vi "make_tilt_stage_array (SubVI).vi"(1 "Tilt settings":T1={"thetaY steps"=0.0, "thetaZ steps"=6.0, "Run thetaY?"=FALSE, "Run thetaZ?"=FALSE, "# repeats \n   in thetaY"=0, "# repeats \n   in thetaZ"=0}) -> (0 "Tot Stage Arr":dbl[][](array[numeric]))   [LabVIEW 2016]
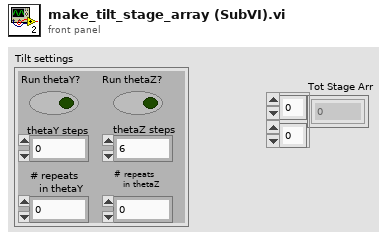
[diagram p1: front panel]
types:
  T1 = cluster{"thetaY steps":dbl, "thetaZ steps":dbl, "Run thetaY?":bool, "Run thetaZ?":bool, "# repeats \n   in thetaY":i32, "# repeats \n   in thetaZ":i32}
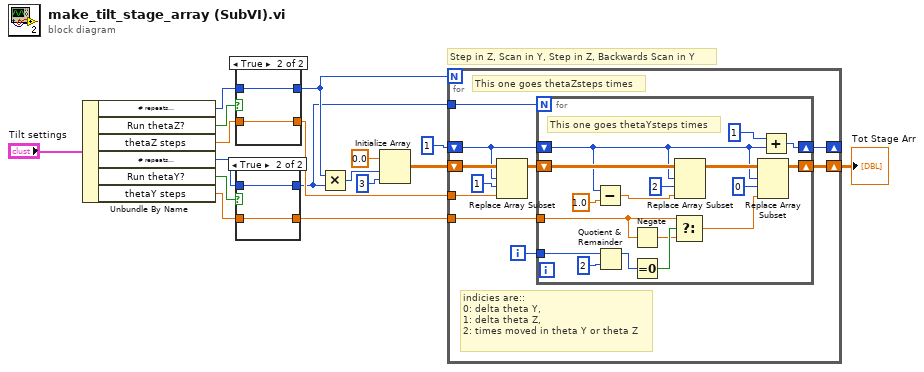
[diagram p0: block diagram]
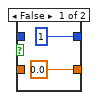
[diagram p2: hidden frame]
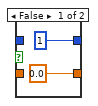
[diagram p3: hidden frame]
diagram:
  # "Step in Z, Scan in Y, Step in Z, Backwards Scan in Y"
  n1 = Unbundle By Name("Tilt settings") -> ("# repeats \n   in thetaZ"=w6:i32, "Run thetaZ?"=w5:bool, "thetaZ steps"=w4:dbl, "# repeats \n   in thetaY"=w9:i32, "Run thetaY?"=w8:bool, "thetaY steps"=w7:dbl)
  n2 = case shown="True" w5 {
    tunnel: w4 -> [_ w20]
    tunnel: w6 -> [_ w21]
    tunnel: [1 ("# steps to\nend thetaY") w21] -> w3
    tunnel: [0.0 ("end thetaZ") w20] -> w12
    frame False {
    }
    frame True {
    }
  }
  n3 = case shown="True" w8 {
    tunnel: w7 -> [_ w24]
    tunnel: w9 -> [_ w25]
    tunnel: [1 ("# steps to\nend thetaY") w25] -> w2
    tunnel: [0.0 ("end thetaZ") w24] -> w11
    frame False {
    }
    frame True {
    }
  }
  n4 = Multiply(x=w3, y=w2) -> (x*y=w1:i32)
  n5 = Initialize Array(0.0 ("element"), w1, 3 ("dimension size")) -> (w10:dbl[][])
  n6 = for {
    N: w3 -> [_]
    tunnel: w11 -> [w35]
    shift-right: [w27] -> _
    shift-left: 1 -> [w29]
    tunnel: w12 -> [w33]
    tunnel: w2 -> [w31]
    shift-right: [w32] -> w13
    shift-left: w10 -> [w30]
    i -> [w28]
    # "indicies are:: \n0: delta theta Y, \n1: delta theta Z, \n2: times moved in theta Y or theta Z"
    # "This one goes thetaZsteps times"
    n7 = Replace Array Subset(array=w30, new element=w33, index (row)=w29, index (col)=1 ("disabled index (col)")) -> (w26:dbl[][])
    n8 = for {
      N: w31 -> [_]
      tunnel: w35 -> [w46]
      tunnel: w28 -> [w45]
      shift-right: [w40] -> w27
      shift-left: w29 -> [w36]
      shift-right: [w44] -> w32
      shift-left: w26 -> [w42]
      # "This one goes thetaYsteps times"
      n9 = Subtract(x=w36, y=1.0) -> (x-y=w38:dbl)
      n10 = Quotient & Remainder(x=w45, y=2) -> (x-y*floor(x/y)=w50:i32)  [unwired: 1 out]
      n11 = Negate(x=w46) -> (-x=w47:dbl)
      n12 = Equal To 0?(x=w50) -> (x = 0?=w51:bool)
      n13 = Select(t=w46, s=w51, f=w47) -> (s? t:f=w48:dbl)
      n14 = Replace Array Subset(array=w42, new element=w38, index (row)=w36, index (col)=2 ("disabled index (col)")) -> (w43:dbl[][])
      n15 = Replace Array Subset(array=w43, new element=w48, index (row)=w36, index (col)=0 ("disabled index (col)")) -> (w44:dbl[][])
      n16 = Add(x=1 ("y"), y=w36) -> (x+y=w40:i32)
    }
  }
  "Tot Stage Arr" <- w13
